vi "Dashboard Global Data.vi"() -> ()   [LabVIEW 2011]
panel:
  in  "Robot IP Address":string
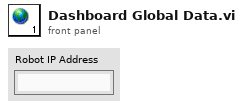
[diagram p1: front panel]
diagram:
